vi "write new operation mode.vi"(8 "error in (no error)":errorcluster, 10 "new operation mode":T1, 11 "CCDCamera in":refnum<class "Sim_CCD.lvclass">) -> (0 "error out":errorcluster, 3 "CCDCamera out":refnum<class "Sim_CCD.lvclass">)   [LabVIEW 2018, in "Sim_CCD.lvclass"]
uses:
  Sim_CCD.lvclass
  Sim_CCD.lvclass/Sim_CCD.ctl
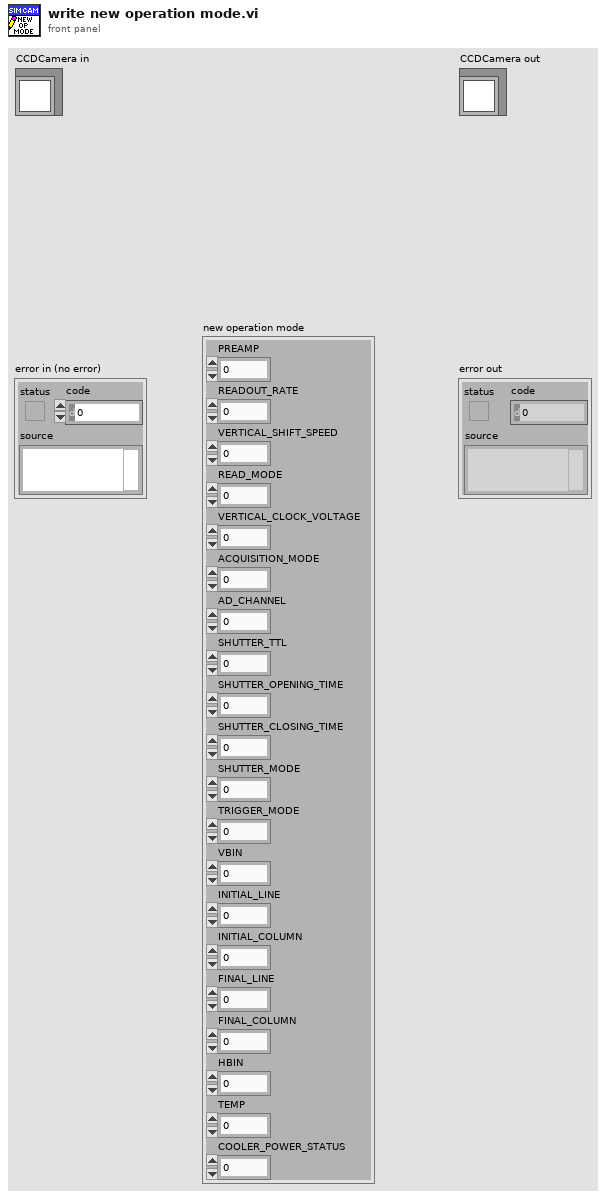
[diagram p1: front panel]
types:
  T1 = cluster{"PREAMP":u16, "READOUT_RATE":u16, "VERTICAL_SHIFT_SPEED":u16, "READ_MODE":u16, "VERTICAL_CLOCK_VOLTAGE":u16, "ACQUISITION_MODE":u16, "AD_CHANNEL":u16, "SHUTTER_TTL":u16, "SHUTTER_OPENING_TIME":u16, "SHUTTER_CLOSING_TIME":u16, "SHUTTER_MODE":u16, "TRIGGER_MODE":u16, "VBIN":u16, "INITIAL_LINE":u16, "INITIAL_COLUMN":u16, "FINAL_LINE":u16, "FINAL_COLUMN":u16, "HBIN":u16, "TEMP":i32, "COOLER_POWER_STATUS":u16}
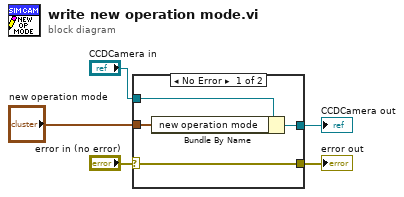
[diagram p0: block diagram]
diagram:
  n1 = case shown="No Error" "error in (no error)" {
    selector: "error in (no error)" -> [w7 w10]
    tunnel: [w7 w10] -> w4
    tunnel: [w9 w11] -> w2
    tunnel: "CCDCamera in" -> [w8 w11]
    tunnel: "new operation mode" -> [w6 _]
    frame No Error {
      n2 = Bundle By Name(cluster=w8, "new operation mode"=w6) -> (w9:refnum<class "Sim_CCD.lvclass">)
    }
    frame Error {
    }
  }
  "error out" <- w4
  "CCDCamera out" <- w2
